vi "New Array Element.vi"(7 "Value Type (String)":T1, 8 "error in (no error)":errorcluster, 11 "Config Element in":refnum<class "Config Element.lvclass">) -> (0 "error out":errorcluster, 1 "Child Index":i32, 2 "New Child":refnum<class "Config Element.lvclass">, 3 "Config Element out":refnum<class "Config Element.lvclass">)   [LabVIEW 2023, in "CDM-Config.lvlib" / "Config Element.lvclass"]
uses:
  Config Element.lvclass
  Value Type.ctl
  Config Element.lvclass/Config Element.ctl
  Config Manager/Config Manager.lvclass
  CDM-Config.lvlib
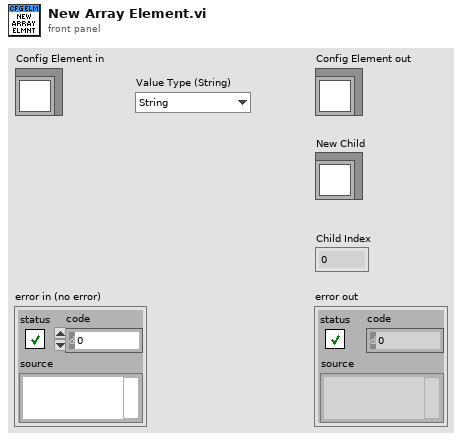
[diagram p1: front panel]
types:
  T1 = typedef "CDM-Config.lvlib/Value Type.ctl" = enum16{"String", "Number", "Bool", "Object", "Array"}
  T2 = typedef "CDM-Config.lvlib/Config Element.lvclass/Element Data.ctl" = cluster{"Node Info":T3, "Owner":refnum<class>, "Changed":bool, "Name":string, "Meta Data":T4[], "Value Type":T1, "Value":variant}
  T3 = typedef "CDM-Config.lvlib/Node Info.ctl" = cluster{"Index":i32, "Parent":i32, "Children":i32[]}
  T4 = typedef "CDM-Config.lvlib/Meta Data.ctl" = cluster{"Name":string, "Value":string}
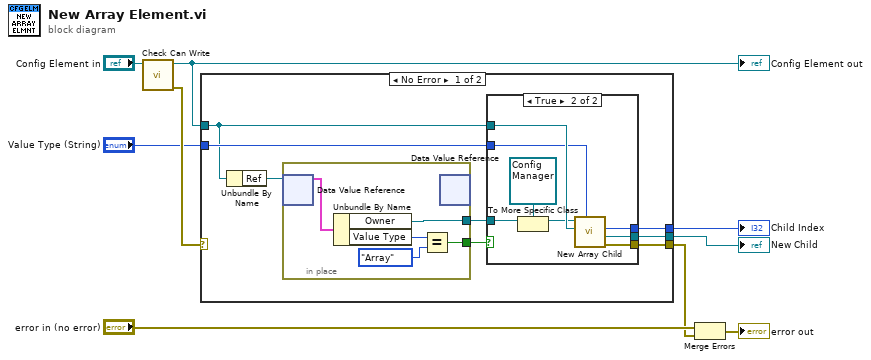
[diagram p0: block diagram]
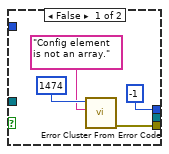
[diagram p2: hidden frame]
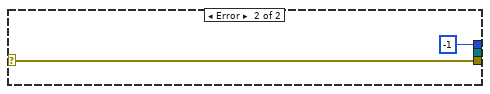
[diagram p3: hidden frame]
diagram:
  n1 = call "Check Can Write.vi"("Config Element in"="Config Element in") -> ("error out"=w9:errorcluster, "Config Element out"=w1:refnum<class "Config Element.lvclass">)  [unwired: 9 in]
  "Config Element out" <- w1
  n2 = case shown="No Error" w9 {
    selector: w9 -> [_ w35]
    tunnel: [w17 _] -> w7
    tunnel: [w16 w35] -> w5
    tunnel: [w15 -1 ("Child Index")] -> w4
    tunnel: "Value Type (String)" -> [w11 _]
    tunnel: w1 -> [w10 _]
    frame No Error {
      n3 = Unbundle By Name(w10) -> ("Ref"=w14:refnum<data-value>)
      n4 = in-place {
        in-place-border: [w33] -> w12
        in-place-border: [w30] -> w13
        n5 = in-place-dvr #1(w14) -> (w34:T2)  [unwired: 1 out]
        n6 = Unbundle By Name(w34) -> ("Owner"=w33:refnum<class>, "Value Type"=w32:T1)
        n7 = Equal?(x=w32, y=Value_Type."Array") -> (x = y?=w30:bool)
        n8 = in-place-dvr #1() -> ()  [unwired: 1 in, 2 out]
      }
      n9 = case shown="True" w13 {
        tunnel: [_ w29] -> w17
        tunnel: [w20 w28] -> w16
        tunnel: [-1 ("Child Index") w27] -> w15
        tunnel: w10 -> [_ w26]
        tunnel: w12 -> [_ w24]
        tunnel: w11 -> [_ w22]
        frame False {
          n10 = call <vilib>:"Error Cluster From Error Code.vi"("error message (\"\")"="Config element is not an array.", "error code (0)"=1474) -> ("error out"=w20:errorcluster)  [unwired: 7 in]
        }
        frame True {
          n11 = To More Specific Class(target class=refnum<class "Config Manager.lvclass"> refnum ("Config Manager in"), reference=w24) -> (specific class reference=w25:refnum<class "Config Manager.lvclass">)  [unwired: 1 in, 1 out]
          n12 = call "New Array Child.vi"("Value Type (String)"=w22, "Array Parent"=w26, "Config Manager in"=w25) -> ("error out"=w28:errorcluster, "New Child"=w29:refnum<class "Config Element.lvclass">, "Child Index"=w27:i32)  [unwired: 5 in, 1 out]
        }
      }
    }
    frame Error {
    }
  }
  "New Child" <- w7
  "Child Index" <- w4
  n13 = Merge Errors("error in (no error)", w5) -> (→"error out":errorcluster)
